vi "VCI Read Err Info.vi"(7 "pErrInfo":T1, 9 "CANIndex":u32, 10 "DevIndex":u32, 11 "DevType":u32) -> (3 "function return":u32, 5 "pErrInfo out":T1)   [LabVIEW 2010, in "ControlCAN.lvlib"]
doc: "unsigned int WINAPI VCI_ReadErrInfo(unsigned int DevType,unsigned int DevIndex,unsigned int CANIndex,PVCI_ERR_INFO pErrInfo);"
uses:
  ControlCAN.lvlib
  ControlCAN/Ginkgo_Driver.dll
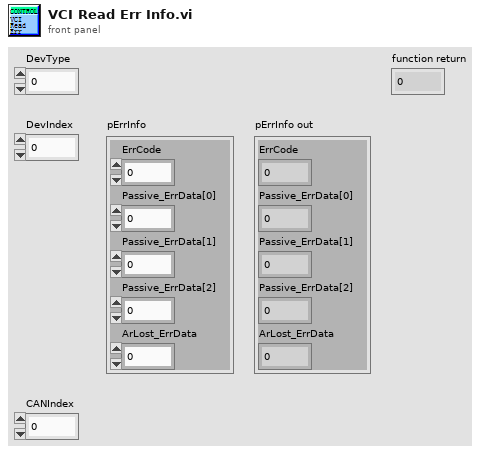
[diagram p1: front panel]
types:
  T1 = cluster{"ErrCode":u32, "Passive_ErrData[0]":u8, "Passive_ErrData[1]":u8, "Passive_ErrData[2]":u8, "ArLost_ErrData":u8}
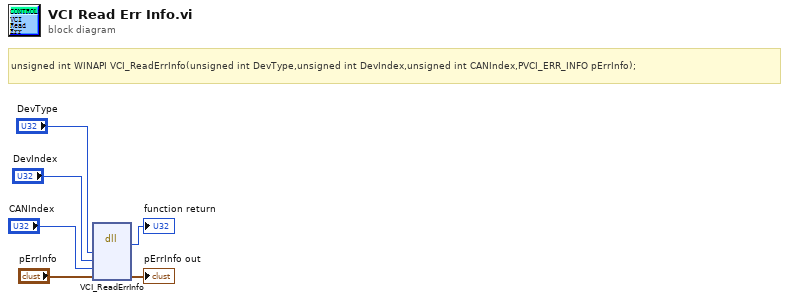
[diagram p0: block diagram]
diagram:
  # "unsigned int WINAPI VCI_ReadErrInfo(unsigned int DevType,unsigned int DevIndex,unsigned int CANIndex,PVCI_ERR_INFO pErrInfo);"
  n1 = dll-call lib="E:/Project/vt_ginkgo/truck/Ginkgo Driver/vs2010/Ginkgo_USB-I2C&SPI&CAN_API_v2.0.3.3/lib/labview_32bit/ControlCAN/Ginkgo_Driver.*" fn="VCI_ReadErrInfo"("DevType"="DevType", "DevIndex"="DevIndex", "CANIndex"="CANIndex", "pErrInfo"="pErrInfo") -> (→"function return":u32, "pErrInfo"=→"pErrInfo out":T1)  [unwired: 6 in, 2 out]
